vi "Configure System.vi"(8 "error in":errorcluster, 9 "Beeper Enabled? (T: On)":bool=TRUE, 10 "Autozero Enabled? (T: On)":bool=TRUE, 11 "VISA resource name":refnum<visa-resource-name>) -> (0 "error out":errorcluster, 3 "VISA resource name out":refnum<visa-resource-name>)   [LabVIEW 2016, in "Keithley 2182A.lvlib"]
uses:
  <instrlib>/Keithley 2182A/Keithley 2182A.lvlib
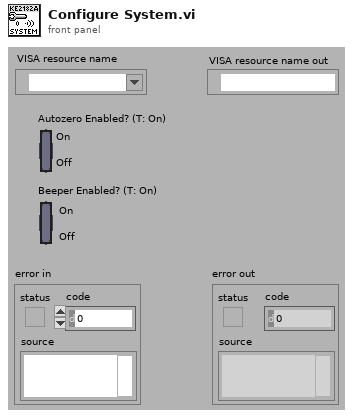
[diagram p1: front panel]
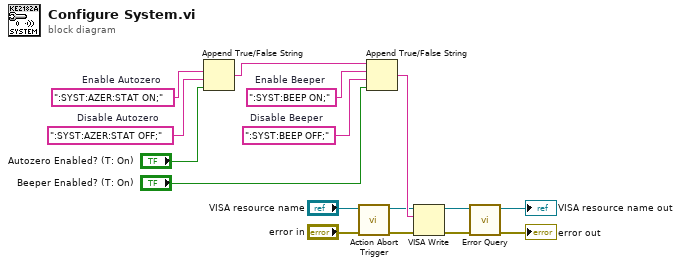
[diagram p0: block diagram]
diagram:
  w12 = ":SYST:BEEP OFF;"  # Disable Beeper
  w11 = ":SYST:BEEP ON;"  # Enable Beeper
  w10 = ":SYST:AZER:STAT OFF;"  # Disable Autozero
  w9 = ":SYST:AZER:STAT ON;"  # Enable Autozero
  n1 = Append True/False String(1:"Autozero Enabled? (T: On)", 2:w10, 3:w9) -> (0:w13:string)  [unwired: 1 in]
  n2 = call <instrlib>:"Action Abort Trigger.vi"("error in"="error in", "VISA resource name"="VISA resource name") -> ("error out"=w6:errorcluster, "VISA resource name out"=w7:refnum<visa-resource-name>)  [unwired: 8 in]
  n3 = Append True/False String(1:"Beeper Enabled? (T: On)", 2:w12, 3:w11, 4:w13) -> (0:w14:string)
  n4 = VISA Write(VISA resource name=w7, write buffer=w14, error in (no error)=w6) -> (VISA resource name out=w4:refnum<visa-resource-name>, error out=w3:errorcluster)  [unwired: 1 out]
  n5 = call <instrlib>:"Error Query.vi"("error in (no error)"=w3, "VISA resource name"=w4) -> ("error out"=→"error out":errorcluster, "VISA resource name out"=→"VISA resource name out":refnum<visa-resource-name>)  [unwired: 6 in, 2 out]
